vi "DB_ConfiguraEquipos.vi"() -> ()   [LabVIEW 2018]
uses:
  <vilib>/RAFA Solutions/Harmony UI Controls Kit/Boolean/OK Button.ctl
  <vilib>/RAFA Solutions/Harmony UI Controls Kit/Boolean/Blank Button - Green.ctl
  <vilib>/RAFA Solutions/Harmony UI Controls Kit/Boolean/Blank Button - Red.ctl
  <vilib>/Utility/miscctls.llb/LVRowAndColumnTypeDef.ctl
  <vilib>/Utility/miscctls.llb/LVBoundsTypeDef.ctl
  <vilib>/event_ctls.llb/eventvkey.ctl
  <vilib>/addons/database/Connection.llb/DB Tools Open Connec (Path).vi
  <vilib>/addons/database/NI_Database_API.lvlib
  <vilib>/RAFA Solutions/Harmony UI Controls Kit/Flat UI Design.lvlib
panel:
  out "no hay equipos":bool
  in  "SALIR":T1
  in  "habilitar":T2
  in  "confirmar":T3
  in  "Tabla de Equipos":i32(listbox)
  in  "DESCRIPCION":string
  in  "NOMBRE_EQUIPO":string
  in  "IP_EQUIPO":string
  in  "ESTADO EQUIPO":string(combo)
  out "Equipos":string[][](table)=[["Select...", "0.00", "This Week", "0.0", "0", "0", "0", "0", "0", "0", "0", "0"], ["Select...", "0.00", "This Week", "0.0", "0", "0", "0", "0", "0", "0", "0", "0"], ["Select...", "0.00", "This Week", "0.0", "0", "0", "0", "0", "0", "0", "0", "0"], ["Select...", "0.00", "This Week", "0.0", "0", "0", "0", "0", "0", "0", "0", "0"], ["Select...", "0.00", "This Week", "0.0", "0", "0", "0", "0", "0", "0", "0", "0"], ["Select...", "0.00", "This Week", "0.0", "0", "0", "0", "0", "0", "0", "0", "0"], ["Select...", "0.00", "This Week", "0.0", "0", "0", "0", "0", "0", "0", "0", "0"], ["Select...", "0.00", "This Week", "0.0", "0", "0", "0", "0", "0", "0", "0", "0"], ["Select...", "0.00", "This Week", "0.0", "0", "0", "0", "0", "0", "0", "0", "0"], ["Select...", "0.00", "This Week", "0.0", "0", "0", "0", "0", "0", "0", "0", "0"], ["Total", "", "", "0", "0", "0", "0", "0", "0", "0", "0", ""]]
  # "Equipos Actuales"
  # "Nueva Configuración de Equipos"
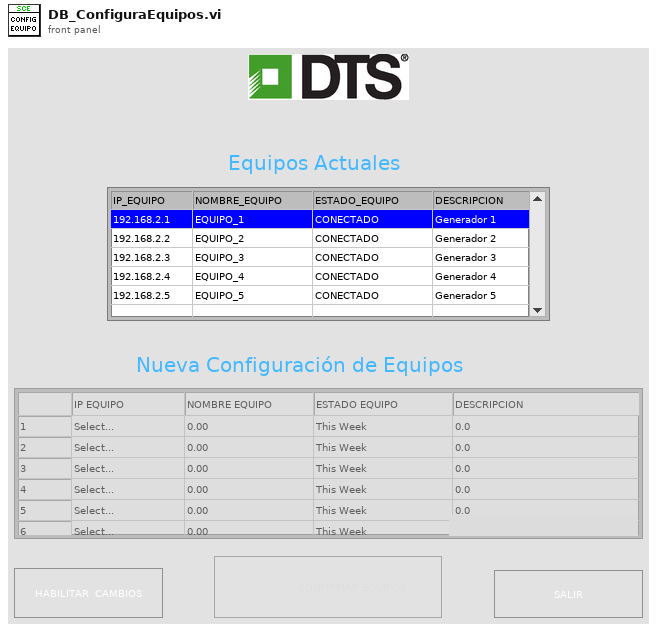
[diagram p1: front panel]
types:
  T1 = typedef "Flat UI Design.lvlib/Blank Button - Red.ctl" = bool
  T2 = typedef "Flat UI Design.lvlib/Blank Button - Green.ctl" = bool
  T3 = typedef "Flat UI Design.lvlib/OK Button.ctl" = bool
  T4 = typedef "LVRowAndColumnTypeDef.ctl" = cluster{"Row":i32, "Column":i32}
  T5 = cluster{"IP_EQUIPO":string, "NOMBRE_EQUIPO":string, "ESTADO_EQUIPO":string, "DESCRIPCION":string}
  T6 = cluster{"IP_EQUIPO":string, "NOMBRE_EQUIPO":string, "ESTADO_EQUIPO":string, "DESCRIPCION":string}[]
  T7 = typedef "LVBoundsTypeDef.ctl" = cluster{"Width":u32, "Height":u32}
  T8 = typedef "eventvkey.ctl" = enum16{"ASCII", "Enter", "Return", "Shift", "Ctrl", "Alt", "Cmd", "Opt", "Caps", "NumLock", "Clear", "Break", "Up", "Down", "Left", "Right", "Insert", "Delete", "Home", "End", "PageUp", "PageDown", "Escape", "Help", "Pause", "ScrollLock", "F1", "F2", "F3", "F4", "F5", "F6", "F7", "F8", "F9", "F10", "F11", "F12", "F13", "F14", "F15", "F16", "F17", "F18", "F19", "F20", "F21", "F22", "F23", "F24", "Play", "VolumeUp", "VolumeDown", "Mute", "Two Byte Char"}
  T9 = enum8{"Enabled", "Disabled", "Disabled and Grayed Out"}
  T10 = typedef "NI_Database_API.lvlib/Conn ObjectReference.ctl" = refnum<k1>
  T11 = typedef "LVPoint32TypeDef.ctl" = cluster{"Horizontal":i32, "Vertical":i32}
  T12 = typedef "LVPositionTypeDef.ctl" = cluster{"Left":i32, "Top":i32}
  T13 = typedef "LVFontTypeDef.ctl" = cluster{"Font Name":string, "Size":u16, "Bold":bool, "Italic":bool, "Underline":bool, "Strikeout":bool, "Color":u32}
  T14 = cluster{"Shift":bool, "Ctrl":bool, "Alt":bool, "Cmd":bool, "Opt":bool}
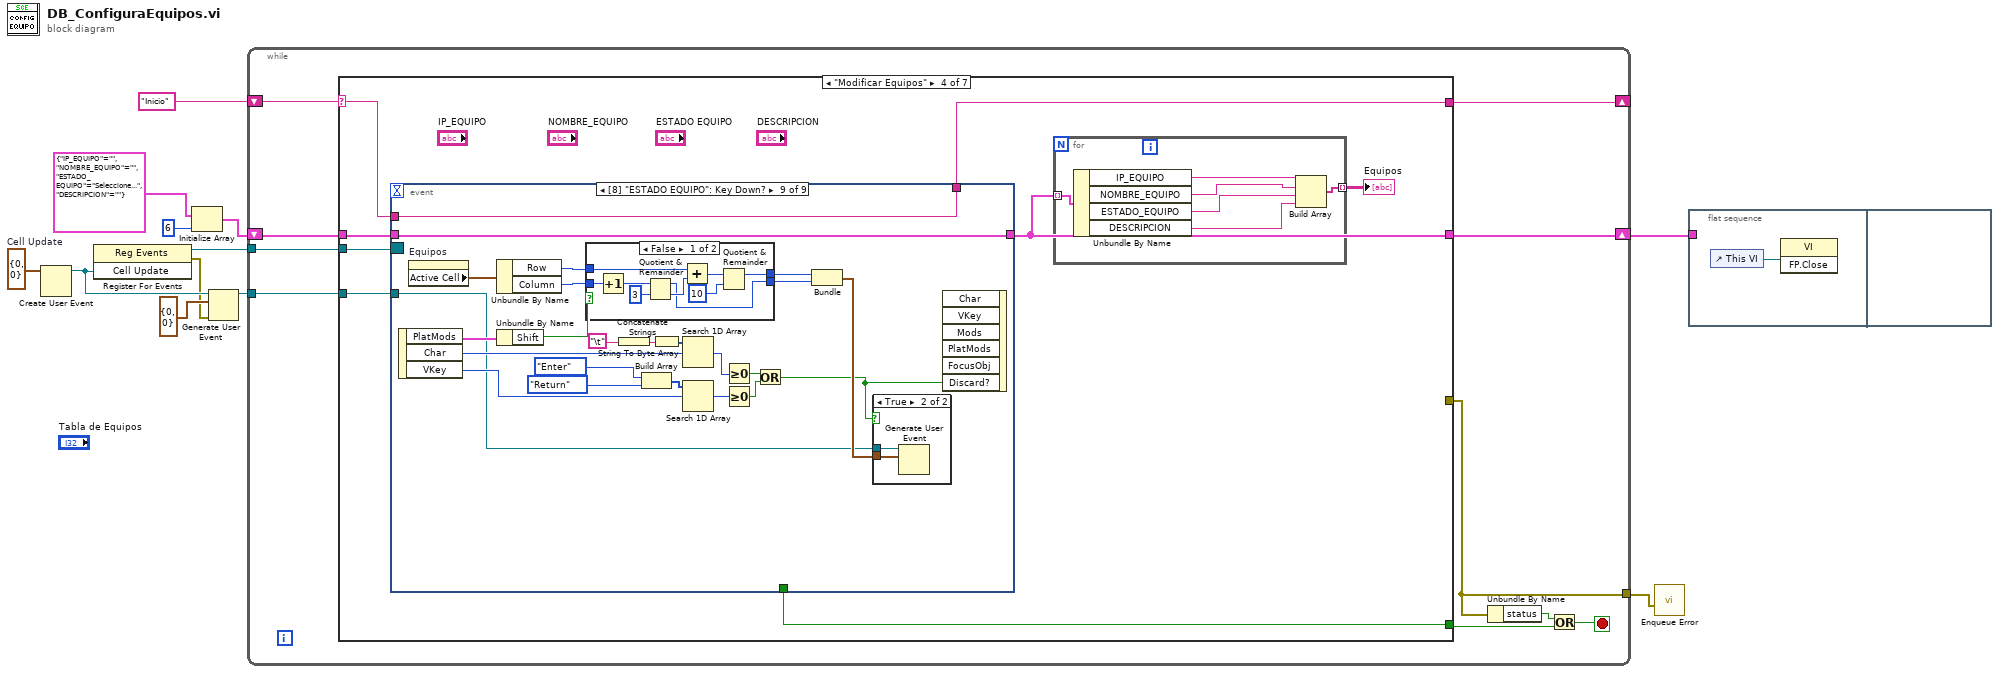
[diagram p0: block diagram]
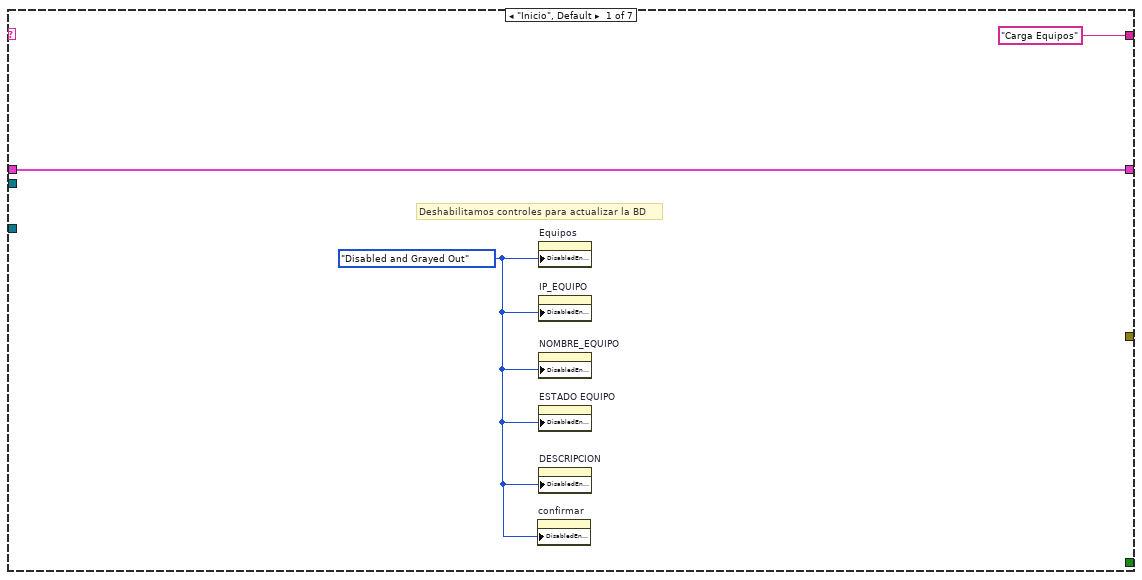
[diagram p2: hidden frame]
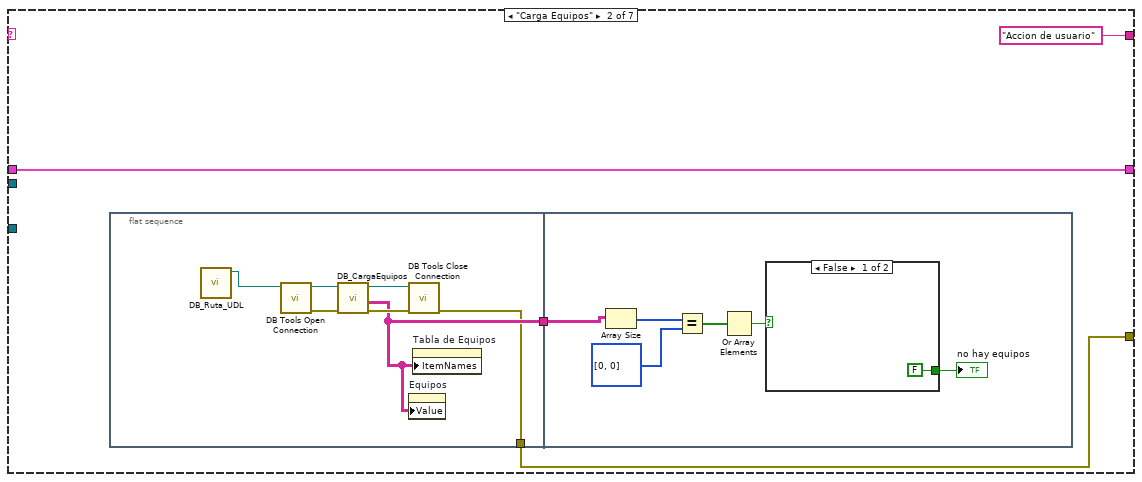
[diagram p3: hidden frame]
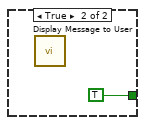
[diagram p4: hidden frame]
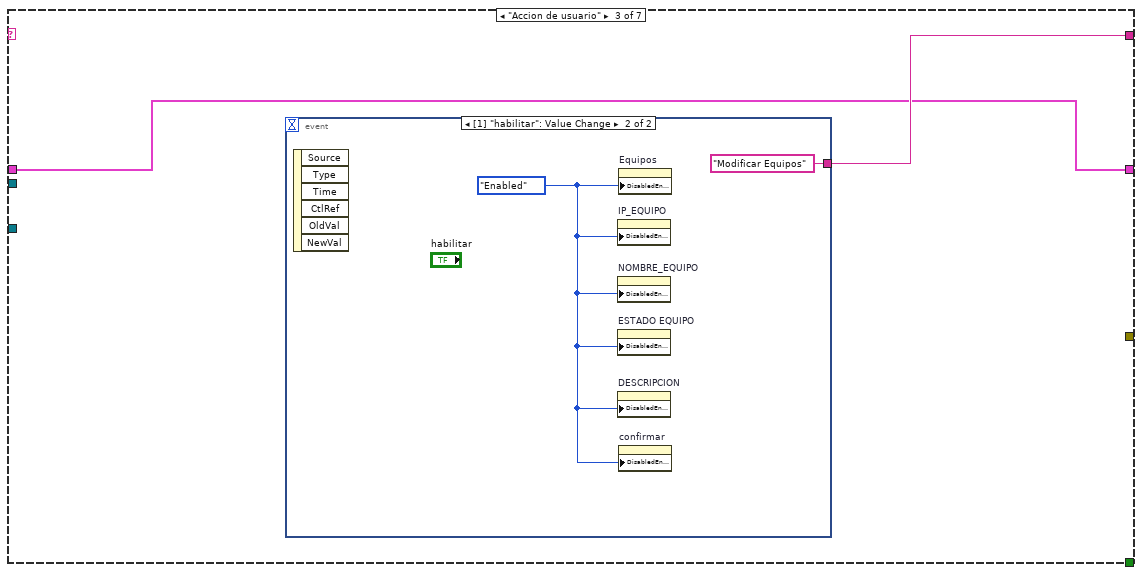
[diagram p5: hidden frame]
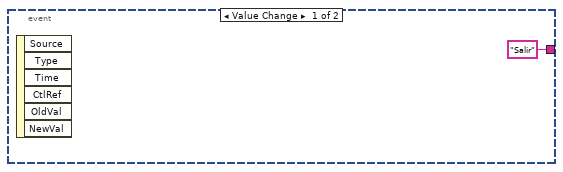
[diagram p6: hidden frame]
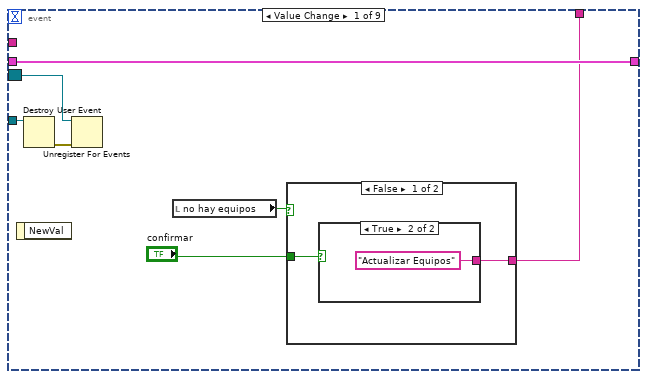
[diagram p7: hidden frame]
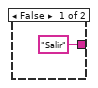
[diagram p8: hidden frame]
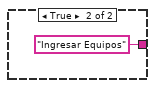
[diagram p9: hidden frame]
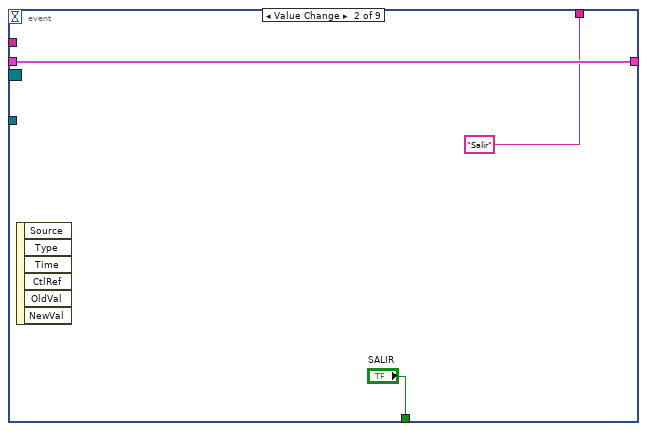
[diagram p10: hidden frame]
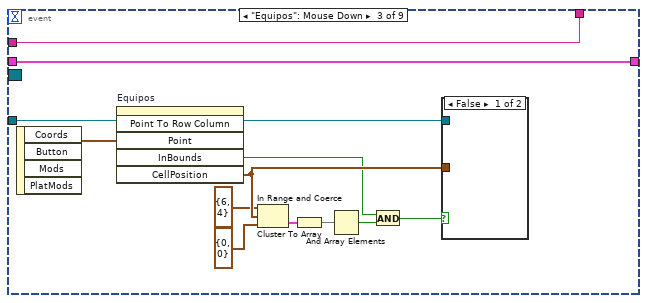
[diagram p11: hidden frame]
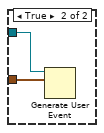
[diagram p12: hidden frame]
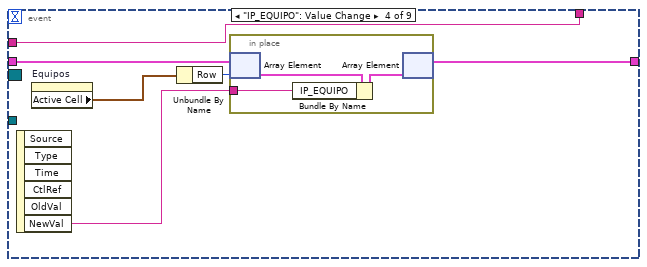
[diagram p13: hidden frame]
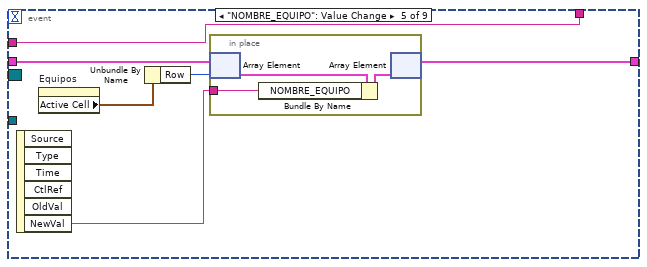
[diagram p14: hidden frame]
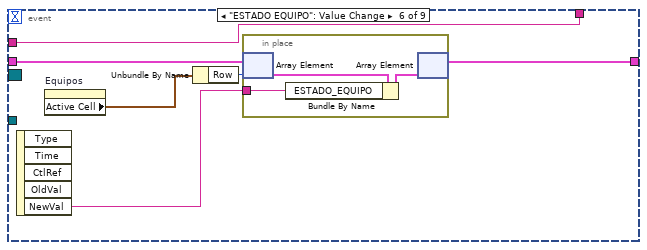
[diagram p15: hidden frame]
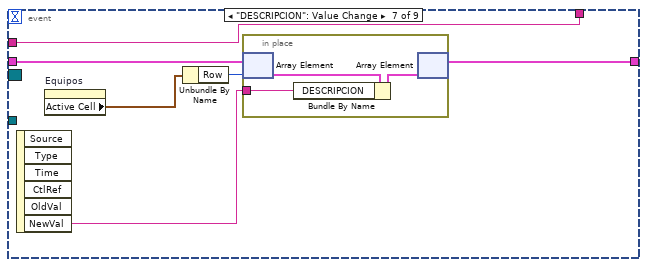
[diagram p16: hidden frame]
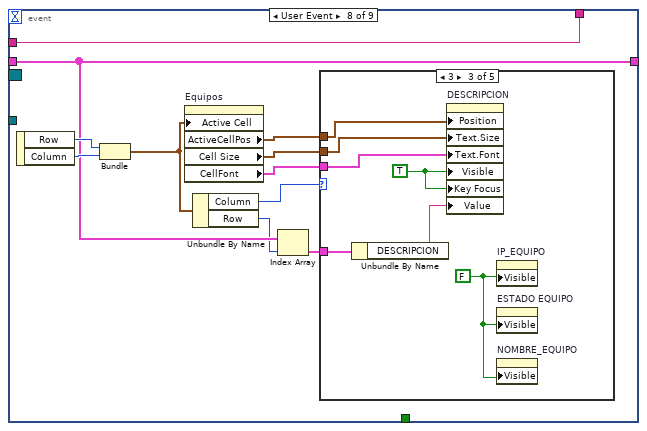
[diagram p17: hidden frame]
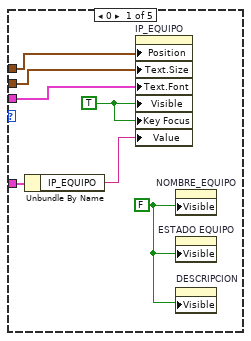
[diagram p18: hidden frame]
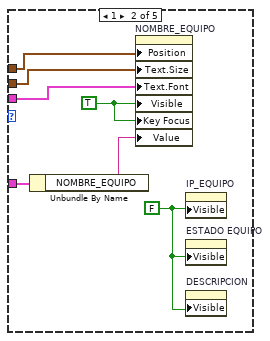
[diagram p19: hidden frame]
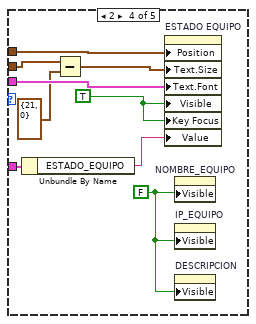
[diagram p20: hidden frame]
diagram:
  w10 = T4 {"Row"=0, "Column"=0}  # Cell Update
  n1 = Create User Event(user event datatype=w10) -> (user event=w8:refnum<user-event>)  [unwired: 1 in, 1 out]
  n2 = register-events(w8) -> (reference out=w9:refnum<event-registration>, error out=w6:errorcluster)  [unwired: 2 in]
  n3 = Initialize Array(T5 {"IP_EQUIPO"="", "NOMBRE_EQUIPO"="", "ESTADO_EQUIPO"="Seleccione...", "DESCRIPCION"=""} ("Dilution Product Selection"), 6 ("dimension size")) -> (w11:T6)
  n4 = Generate User Event(user event=w8, event data cluster=T4 {"Row"=0, "Column"=0} ("event data"), error in=w6) -> (user event out=w5:refnum<user-event>)  [unwired: 1 in, 1 out]
  n5 = while {
    shift-right: [w20] -> w2
    shift-left: w11 -> [w22]
    tunnel: w9 -> [w21]
    tunnel: w5 -> [w19]
    shift-right: [w17] -> _
    shift-left: "Inicio" -> [w18]
    tunnel: [w13] -> w1
    stop <- w16 stop-if-true
    n6 = case shown="\"Modificar Equipos\"" w18 {
      selector: w18 -> [_ _ _ w50 _ _ _]
      tunnel: [_ _ _ w49 _ _ TRUE ("Dilute")] -> w15
      tunnel: w22 -> [w25 w29 w44 w56 w219 w229 w235]
      tunnel: w21 -> [_ _ _ w55 _ _ _]
      tunnel: [w25 w29 w44 w54 w219 w229 w235] -> w20
      tunnel: w19 -> [_ _ _ w53 _ _ _]
      tunnel: ["Carga Equipos" "Accion de usuario" w45 w51 "Salir" "Salir" ""] -> w17
      tunnel: [_ w26 _ _ w213 w223 _] -> w13
      frame "Inicio", Default {
        w23 = T9."Disabled and Grayed Out" ("Disabled")
        # "Deshabilitamos controles para actualizar la BD"
        n7 = property on="confirmar" class="Bool"("DisabledEnum"=w23) -> ()  [unwired: 2 in, 2 out]
        n8 = property on="Equipos" class="Tbl (strict)"("DisabledEnum"=w23) -> ()  [unwired: 2 in, 2 out]
        n9 = property on="IP_EQUIPO" class="Str"("DisabledEnum"=w23) -> ()  [unwired: 2 in, 2 out]
        n10 = property on="NOMBRE_EQUIPO" class="Str"("DisabledEnum"=w23) -> ()  [unwired: 2 in, 2 out]
        n11 = property on="ESTADO EQUIPO" class="CmbBox"("DisabledEnum"=w23) -> ()  [unwired: 2 in, 2 out]
        n12 = property on="DESCRIPCION" class="Str"("DisabledEnum"=w23) -> ()  [unwired: 2 in, 2 out]
      }
      frame "Carga Equipos" {
        n13 = flat-sequence {
          tunnel: [w31] -> w27
          tunnel: [w30] -> w26
          tunnel: w27 -> [w36]
          frame #0 {
            n14 = call "DB_Ruta_UDL.vi"() -> ("UDL ruta"=w32:path)  [unwired: 11 in]
            n15 = call-poly <vilib>:"DB Tools Open Connection.vi"("connection information"=w32) -> ("error out"=w35:errorcluster, "connection reference"=w34:T10)  [unwired: 7 in]
            n16 = call "DB_CargaEquipos.vi"("error in (no error)"=w35, "db in"=w34) -> ("error out"=w33:errorcluster, "Equipos"=w31:string[][])  [unwired: 2 in, 6 out]
            n17 = call <vilib>:"DB Tools Close Connection.vi"("error in (no error)"=w33, "connection reference"=w34) -> ("error out"=w30:errorcluster)  [unwired: 5 in]
            n18 = property on="Equipos" class="Tbl (strict)"("Value"=w31) -> ()  [unwired: 2 in, 2 out]
            n19 = property on="Tabla de Equipos" class="MCListbox (strict)"("ItemNames"=w31) -> ()  [unwired: 2 in, 2 out]
          }
          frame #1 {
            n20 = Array Size(array=w36) -> (size(s)=w41:i32[])
            n21 = Equal?(x=w41, y=i32[] [0, 0]) -> (x = y?=w38:bool[])
            n22 = Or Array Elements(Boolean array=w38) -> (logical OR=w39:bool)
            n23 = case shown="False" w39 {
              tunnel: [FALSE TRUE] -> w37
              frame False {
              }
              frame True {
                n24 = call "Display Message to User"() -> ()  [unwired: 10 in, 2 out]
              }
            }
            "no hay equipos" <- w37
          }
        }
      }
      frame "Accion de usuario" {
        n25 = event shown="[1] \"habilitar\": Value Change" {
          selector: _ -> [_ _]
          dyn-events: _ -> [_ _]
          timeout: _ -> [_ _]
          tunnel: ["Salir" "Modificar Equipos"] -> w45
          event Value Change {
            n26 = event-data() -> ()  [unwired: 1 in, 6 out]
          }
          event Value Change {
            w47 = T9."Enabled" ("Disabled")
            n27 = event-data() -> ()  [unwired: 1 in, 6 out]
            n28 = property on="IP_EQUIPO" class="Str"("DisabledEnum"=w47) -> ()  [unwired: 2 in, 2 out]
            n29 = property on="NOMBRE_EQUIPO" class="Str"("DisabledEnum"=w47) -> ()  [unwired: 2 in, 2 out]
            n30 = property on="ESTADO EQUIPO" class="CmbBox"("DisabledEnum"=w47) -> ()  [unwired: 2 in, 2 out]
            n31 = property on="DESCRIPCION" class="Str"("DisabledEnum"=w47) -> ()  [unwired: 2 in, 2 out]
            n32 = property on="Equipos" class="Tbl (strict)"("DisabledEnum"=w47) -> ()  [unwired: 2 in, 2 out]
            n33 = property on="confirmar" class="Bool"("DisabledEnum"=w47) -> ()  [unwired: 2 in, 2 out]
          }
        }
      }
      frame "Modificar Equipos" {
        n34 = event shown="[8] \"ESTADO EQUIPO\": Key Down?" {
          selector: w55 -> [w67 _ _ _ _ _ _ _ _]
          dyn-events: _ -> [_ _ _ _ _ _ _ _ _]
          timeout: _ -> [_ _ _ _ _ _ _ _ _]
          tunnel: w56 -> [w69 w77 w80 w97 w106 w115 w124 w131 w192]
          tunnel: [w69 w77 w80 w95 w104 w113 w122 w131 w192] -> w54
          tunnel: w53 -> [w68 _ w79 _ _ _ _ _ w170]
          tunnel: [w64 "Salir" w78 w92 w101 w110 w119 w128 w169] -> w51
          tunnel: w50 -> [_ _ w78 w92 w101 w110 w119 w128 w169]
          tunnel: [_ "SALIR" _ _ _ _ _ _ _] -> w49
          event Value Change {
            n35 = event-data() -> ()  [unwired: 1 in, 1 out]
            n36 = Destroy User Event(user event=w68) -> (error out=w66:errorcluster)  [unwired: 1 in]
            n37 = Unregister For Events(event registration refnum=w67, error in=w66) -> ()  [unwired: 1 out]
            n38 = local read "no hay equipos"() -> (w65:bool)
            n39 = case shown="False" w65 {
              tunnel: [w71 "Ingresar Equipos"] -> w64
              tunnel: "confirmar" -> [w70 _]
              frame False {
                n40 = case shown="True" w70 {
                  tunnel: ["Salir" "Actualizar Equipos"] -> w71
                  frame False {
                  }
                  frame True {
                  }
                }
              }
              frame True {
              }
            }
          }
          event Value Change {
            n41 = event-data() -> ()  [unwired: 1 in, 6 out]
          }
          event "Equipos": Mouse Down {
            n42 = event-data() -> ("Coords"=w89:T11)  [unwired: 1 in, 3 out]
            n43 = invoke on="Equipos" class="Tbl (strict)" method="Point To Row Column"("Point"=w89) -> ("InBounds"=w84:bool, "CellPosition"=w88:T4)  [unwired: 5 in, 4 out]
            n44 = In Range and Coerce(upper limit=T4 {"Row"=6, "Column"=4}, x=w88, lower limit=T4 {"Row"=0, "Column"=0}) -> (In Range?=w85:cluster{"Row":bool, "Column":bool})  [unwired: 1 out]
            n45 = Cluster To Array(cluster=w85) -> (array=w82:bool[])
            n46 = And Array Elements(Boolean array=w82) -> (logical AND=w81:bool)
            n47 = And(x=w84, y=w81) -> (x .and. y?=w83:bool)
            n48 = case shown="False" w83 {
              tunnel: w88 -> [_ w91]
              tunnel: w79 -> [_ w90]
              frame False {
              }
              frame True {
                n49 = Generate User Event(user event=w90, event data cluster=w91) -> ()  [unwired: 2 in, 2 out]
              }
            }
          }
          event "IP_EQUIPO": Value Change {
            n50 = event-data() -> ("NewVal"=w93:string)  [unwired: 1 in, 5 out]
            n51 = property on="Equipos" class="Tbl (strict)"() -> ("Active Cell"=w94:T4)  [unwired: 2 in, 2 out]
            n52 = Unbundle By Name(w94) -> ("Row"=w96:i32)
            n53 = in-place {
              in-place-border: w93 -> [w98]
              n54 = in-place-array #1(w97, w96) -> (w100:T5)
              n55 = Bundle By Name(cluster=w100, "IP_EQUIPO"=w98) -> (w99:T5)
              n56 = in-place-array #1(w99) -> (w95:T6)  [unwired: 1 out]
            }
          }
          event "NOMBRE_EQUIPO": Value Change {
            n57 = event-data() -> ("NewVal"=w102:string)  [unwired: 1 in, 5 out]
            n58 = property on="Equipos" class="Tbl (strict)"() -> ("Active Cell"=w103:T4)  [unwired: 2 in, 2 out]
            n59 = Unbundle By Name(w103) -> ("Row"=w105:i32)
            n60 = in-place {
              in-place-border: w102 -> [w107]
              n61 = in-place-array #2(w106, w105) -> (w109:T5)
              n62 = Bundle By Name(cluster=w109, "NOMBRE_EQUIPO"=w107) -> (w108:T5)
              n63 = in-place-array #2(w108) -> (w104:T6)  [unwired: 1 out]
            }
          }
          event "ESTADO EQUIPO": Value Change {
            n64 = event-data() -> ("NewVal"=w112:string)  [unwired: 1 in, 4 out]
            n65 = property on="Equipos" class="Tbl (strict)"() -> ("Active Cell"=w111:T4)  [unwired: 2 in, 2 out]
            n66 = Unbundle By Name(w111) -> ("Row"=w114:i32)
            n67 = in-place {
              in-place-border: w112 -> [w116]
              n68 = in-place-array #3(w115, w114) -> (w118:T5)
              n69 = Bundle By Name(cluster=w118, "ESTADO_EQUIPO"=w116) -> (w117:T5)
              n70 = in-place-array #3(w117) -> (w113:T6)  [unwired: 1 out]
            }
          }
          event "DESCRIPCION": Value Change {
            n71 = event-data() -> ("NewVal"=w120:string)  [unwired: 1 in, 5 out]
            n72 = property on="Equipos" class="Tbl (strict)"() -> ("Active Cell"=w121:T4)  [unwired: 2 in, 2 out]
            n73 = Unbundle By Name(w121) -> ("Row"=w123:i32)
            n74 = in-place {
              in-place-border: w120 -> [w125]
              n75 = in-place-array #4(w124, w123) -> (w127:T5)
              n76 = Bundle By Name(cluster=w127, "DESCRIPCION"=w125) -> (w126:T5)
              n77 = in-place-array #4(w126) -> (w122:T6)  [unwired: 1 out]
            }
          }
          event User Event {
            n78 = event-data() -> ("Row"=w138:i32, "Column"=w137:i32)  [unwired: 1 in]
            n79 = Bundle("Row"=w138, "Column"=w137) -> (w132:cluster{"Row":i32, "Column":i32})  [unwired: 1 in]
            n80 = property on="Equipos" class="Tbl (strict)"("Active Cell"=w132) -> ("ActiveCellPos"=w136:T12, "Cell Size"=w135:T7, "CellFont"=w133:T13)  [unwired: 2 in, 2 out]
            n81 = Unbundle By Name(w132) -> ("Column"=w134:i32, "Row"=w130:i32)
            n82 = Index Array(array=w131, index=w130) -> (element=w129:T5)
            n83 = case shown="3" w134 {
              tunnel: w136 -> [w142 w149 w156 w168 _]
              tunnel: w135 -> [w139 w146 w153 w163 _]
              tunnel: w133 -> [w141 w148 w155 w167 _]
              tunnel: w129 -> [w143 w150 w157 w162 _]
              frame 0 {
                w140 = FALSE ("Visible")
                w145 = TRUE ("Key Focus")
                n84 = Unbundle By Name(w143) -> ("IP_EQUIPO"=w144:string)
                n85 = property on="IP_EQUIPO" class="Str"("Position"=w142, "Text.Size"=w139, "Text.Font"=w141, "Visible"=w145, "Key Focus"=w145, "Value"=w144) -> ()  [unwired: 2 in, 2 out]
                n86 = property on="NOMBRE_EQUIPO" class="Str"("Visible"=w140) -> ()  [unwired: 2 in, 2 out]
                n87 = property on="ESTADO EQUIPO" class="CmbBox"("Visible"=w140) -> ()  [unwired: 2 in, 2 out]
                n88 = property on="DESCRIPCION" class="Str"("Visible"=w140) -> ()  [unwired: 2 in, 2 out]
              }
              frame 1 {
                w147 = FALSE ("Visible")
                w152 = TRUE ("Key Focus")
                n89 = Unbundle By Name(w150) -> ("NOMBRE_EQUIPO"=w151:string)
                n90 = property on="NOMBRE_EQUIPO" class="Str"("Position"=w149, "Text.Size"=w146, "Text.Font"=w148, "Visible"=w152, "Key Focus"=w152, "Value"=w151) -> ()  [unwired: 2 in, 2 out]
                n91 = property on="IP_EQUIPO" class="Str"("Visible"=w147) -> ()  [unwired: 2 in, 2 out]
                n92 = property on="ESTADO EQUIPO" class="CmbBox"("Visible"=w147) -> ()  [unwired: 2 in, 2 out]
                n93 = property on="DESCRIPCION" class="Str"("Visible"=w147) -> ()  [unwired: 2 in, 2 out]
              }
              frame 3 {
                w154 = FALSE ("Visible")
                w159 = TRUE ("Key Focus")
                n94 = Unbundle By Name(w157) -> ("DESCRIPCION"=w158:string)
                n95 = property on="DESCRIPCION" class="Str"("Position"=w156, "Text.Size"=w153, "Text.Font"=w155, "Visible"=w159, "Key Focus"=w159, "Value"=w158) -> ()  [unwired: 2 in, 2 out]
                n96 = property on="IP_EQUIPO" class="Str"("Visible"=w154) -> ()  [unwired: 2 in, 2 out]
                n97 = property on="ESTADO EQUIPO" class="CmbBox"("Visible"=w154) -> ()  [unwired: 2 in, 2 out]
                n98 = property on="NOMBRE_EQUIPO" class="Str"("Visible"=w154) -> ()  [unwired: 2 in, 2 out]
              }
              frame 2 {
                w160 = FALSE ("Visible")
                w166 = TRUE ("Key Focus")
                n99 = Unbundle By Name(w162) -> ("ESTADO_EQUIPO"=w161:string)
                n100 = Subtract(x=w163, y=T7 {"Width"=21, "Height"=0} ("x")) -> (x-y=w164:T7)
                n101 = property on="ESTADO EQUIPO" class="CmbBox"("Position"=w168, "Text.Size"=w164, "Text.Font"=w167, "Visible"=w166, "Key Focus"=w166, "Value"=w161) -> ()  [unwired: 2 in, 2 out]
                n102 = property on="NOMBRE_EQUIPO" class="Str"("Visible"=w160) -> ()  [unwired: 2 in, 2 out]
                n103 = property on="IP_EQUIPO" class="Str"("Visible"=w160) -> ()  [unwired: 2 in, 2 out]
                n104 = property on="DESCRIPCION" class="Str"("Visible"=w160) -> ()  [unwired: 2 in, 2 out]
              }
              frame Default {
              }
            }
          }
          event "ESTADO EQUIPO": Key Down? {
            n105 = event-data() -> ("PlatMods"=w171:T14, "Char"=w179:i16, "VKey"=w175:T8)  [unwired: 1 in]
            n106 = property on="Equipos" class="Tbl (strict)"() -> ("Active Cell"=w185:T4)  [unwired: 2 in, 2 out]
            n107 = Unbundle By Name(w185) -> ("Row"=w190:i32, "Column"=w191:i32)
            n108 = Unbundle By Name(w171) -> ("Shift"=w186:bool)
            n109 = case shown="False" w186 {
              tunnel: w191 -> [w203 w212]
              tunnel: w190 -> [w199 w208]
              tunnel: [w196 w205] -> w189
              tunnel: [w195 w204] -> w188
              frame False {
                n110 = Increment(x=w203) -> (x+1=w202:i32)
                n111 = Quotient & Remainder(x=w202, y=3) -> (x-y*floor(x/y)=w195:i32, floor(x/y)=w200:i32)
                n112 = Add(x=w199, y=w200) -> (x+y=w198:i32)
                n113 = Quotient & Remainder(x=w198, y=10) -> (x-y*floor(x/y)=w196:i32)  [unwired: 1 out]
              }
              frame True {
                n114 = Decrement(x=w212) -> (x-1=w211:i32)
                n115 = Quotient & Remainder(x=w211, y=3) -> (x-y*floor(x/y)=w204:i32, floor(x/y)=w209:i32)
                n116 = Add(x=w208, y=w209) -> (x+y=w207:i32)
                n117 = Quotient & Remainder(x=w207, y=10) -> (x-y*floor(x/y)=w205:i32)  [unwired: 1 out]
              }
            }
            n118 = Concatenate Strings("\t") -> (w183:string)
            n119 = Build Array(eventvkey."Enter" ("VKey"), eventvkey."Return" ("VKey")) -> (w176:T8[])
            n120 = String To Byte Array(string=w183) -> (unsigned byte array=w182:u8[])
            n121 = Search 1D Array(1D array=w182, element=w179) -> (index of element=w181:i32)  [unwired: 1 in]
            n122 = Search 1D Array(1D array=w176, element=w175) -> (index of element=w174:i32)  [unwired: 1 in]
            n123 = Greater Or Equal To 0?(x=w181) -> (x >= 0?=w180:bool)
            n124 = Greater Or Equal To 0?(x=w174) -> (x >= 0?=w172:bool)
            n125 = Or(x=w180, y=w172) -> (x .or. y?=w173:bool)
            n126 = Bundle(w189, w188) -> (w187:cluster{i32, i32})  [unwired: 1 in]
            n127 = case shown="True" w173 {
              tunnel: w187 -> [_ w194]
              tunnel: w170 -> [_ w193]
              frame False {
              }
              frame True {
                n128 = Generate User Event(user event=w193, event data cluster=w194) -> ()  [unwired: 2 in, 2 out]
              }
            }
            n129 = event-data("Discard?"=w173) -> ()  [unwired: 6 in, 1 out]
          }
        }
        n130 = for {
          tunnel: [w62] -> w52 mode=indexing
          tunnel: w54 -> [w61] mode=indexing
          n131 = Unbundle By Name(w61) -> ("IP_EQUIPO"=w60:string, "NOMBRE_EQUIPO"=w59:string, "ESTADO_EQUIPO"=w57:string, "DESCRIPCION"=w58:string)
          n132 = Build Array(w60, w59, w57, w58) -> (w62:string[])
        }
        "Equipos" <- w52
      }
      frame "Ingresar Equipos" {
        n133 = property on="Equipos" class="Tbl (strict)"() -> ("Value"=w214:string[][])  [unwired: 2 in, 2 out]
        n134 = call "DB_EscribeTablaEquipos.vi"("Equipos"=w214) -> ("error out"=w217:errorcluster)  [unwired: 9 in, 1 out]
        n135 = Unbundle By Name(w217) -> ("status"=w216:bool)
        n136 = case shown="True" w216 {
          tunnel: ["Configuracion de equipos exitosa" "Configuracion de equipos con errores"] -> w215
          frame False {
            n137 = call "Display Message to User2"("Enable"=TRUE) -> ()  [unwired: 9 in, 2 out]
          }
          frame True {
            n138 = call "Display Message to User5"() -> ()  [unwired: 10 in, 2 out]
          }
        }
        n139 = call "DB_EscribeTablaEventos.vi"("DESCRIPCION"=w215) -> ("error out"=w213:errorcluster)  [unwired: 10 in]
      }
      frame "Actualizar Equipos" {
        n140 = property on="Equipos" class="Tbl (strict)"() -> ("Value"=w224:string[][])  [unwired: 2 in, 2 out]
        n141 = call "DB_ActualizaTablaEquipos.vi"("Equipos"=w224) -> ("error out"=w227:errorcluster)  [unwired: 10 in]
        n142 = Unbundle By Name(w227) -> ("status"=w226:bool)
        n143 = case shown="False" w226 {
          tunnel: ["Actualización de equipos exitosa" "Actualización de equipos con errores"] -> w225
          frame False {
            n144 = call "Display Message to User6"("Enable"=TRUE) -> ()  [unwired: 9 in, 2 out]
          }
          frame True {
            n145 = call "Display Message to User3"("Enable"=TRUE) -> ()  [unwired: 9 in, 2 out]
          }
        }
        n146 = call "DB_EscribeTablaEventos.vi"("DESCRIPCION"=w225) -> ("error out"=w223:errorcluster)  [unwired: 10 in]
      }
      frame "Salir" {
      }
    }
    n147 = Unbundle By Name(w13) -> ("status"=w14:bool)
    n148 = Or(x=w14, y=w15) -> (x .or. y?=w16:T1)
  }
  n149 = call "Enqueue Error.vi"("error in"=w1) -> ()  [unwired: 9 in, 2 out]
  n150 = flat-sequence {
    tunnel: w2 -> [_]
    frame #0 {
      n151 = control-ref of="This VI"() -> (w237:refnum<vi>)
      n152 = invoke class="VI" method="FP.Close"(reference=w237) -> ()  [unwired: 2 in, 3 out]
    }
    frame #1 {
    }
  }
